vi "Read Error.vi"(8 "error in (no error)":errorcluster, 11 "TDMS-Data in":refnum<class "TDMS-Data.lvclass">) -> (0 "error out":errorcluster, 2 "Error":errorcluster, 3 "TDMS-Data out":refnum<class "TDMS-Data.lvclass">)   [LabVIEW 2017, in "BNT_TDMS.lvlib" / "TDMS-Data.lvclass"]
uses:
  TDMS-Data.lvclass
  TDMS-Data.lvclass/TDMS-Data.ctl
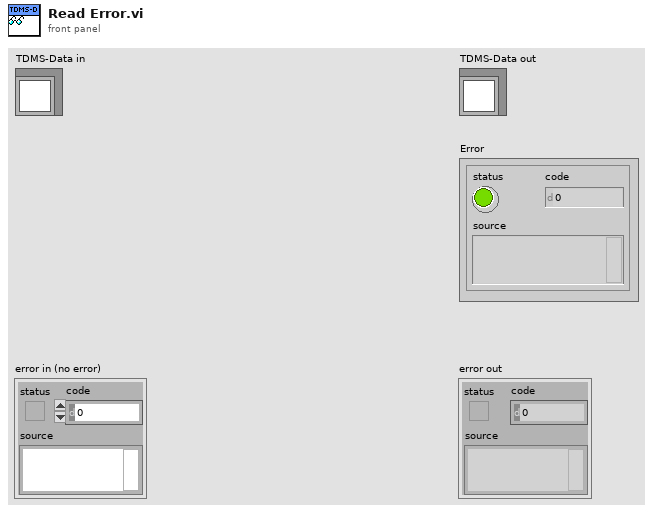
[diagram p1: front panel]
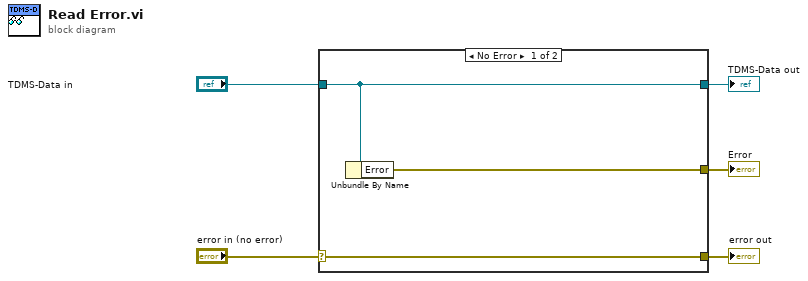
[diagram p0: block diagram]
diagram:
  n1 = case shown="No Error" "error in (no error)" {
    selector: "error in (no error)" -> [w8 w9]
    tunnel: [w8 w9] -> w4
    tunnel: [w7 w10] -> w2
    tunnel: "TDMS-Data in" -> [w7 w10]
    tunnel: [w6 _] -> w1
    frame No Error {
      n2 = Unbundle By Name(w7) -> ("Error"=w6:errorcluster)
    }
    frame Error {
    }
  }
  "error out" <- w4
  "TDMS-Data out" <- w2
  "Error" <- w1
